vi "test_display.vi"() -> ()   [LabVIEW 2016]
uses:
  <vilib>/Utility/miscctls.llb/LVBoundsTypeDef.ctl
panel:
  out "Bounds":T1
  in  "[user-specified font]":T2={"Font Name:"="", "Size"=12, "Strikeout?"=FALSE, "Italic?"=FALSE, "Underline?"=FALSE, "Outline?"=FALSE, "Shadow?"=FALSE, "Bold?"=FALSE}
  in  "desired font(Application)":T3(ring)=enum."Application Font"
  in  "OK Button":bool
  in  "stop":bool
  out "text":string
  in  "origin":cluster{"x":i16, "y":i16}
  in  "alignment":T4
  out "2D Picture":picture
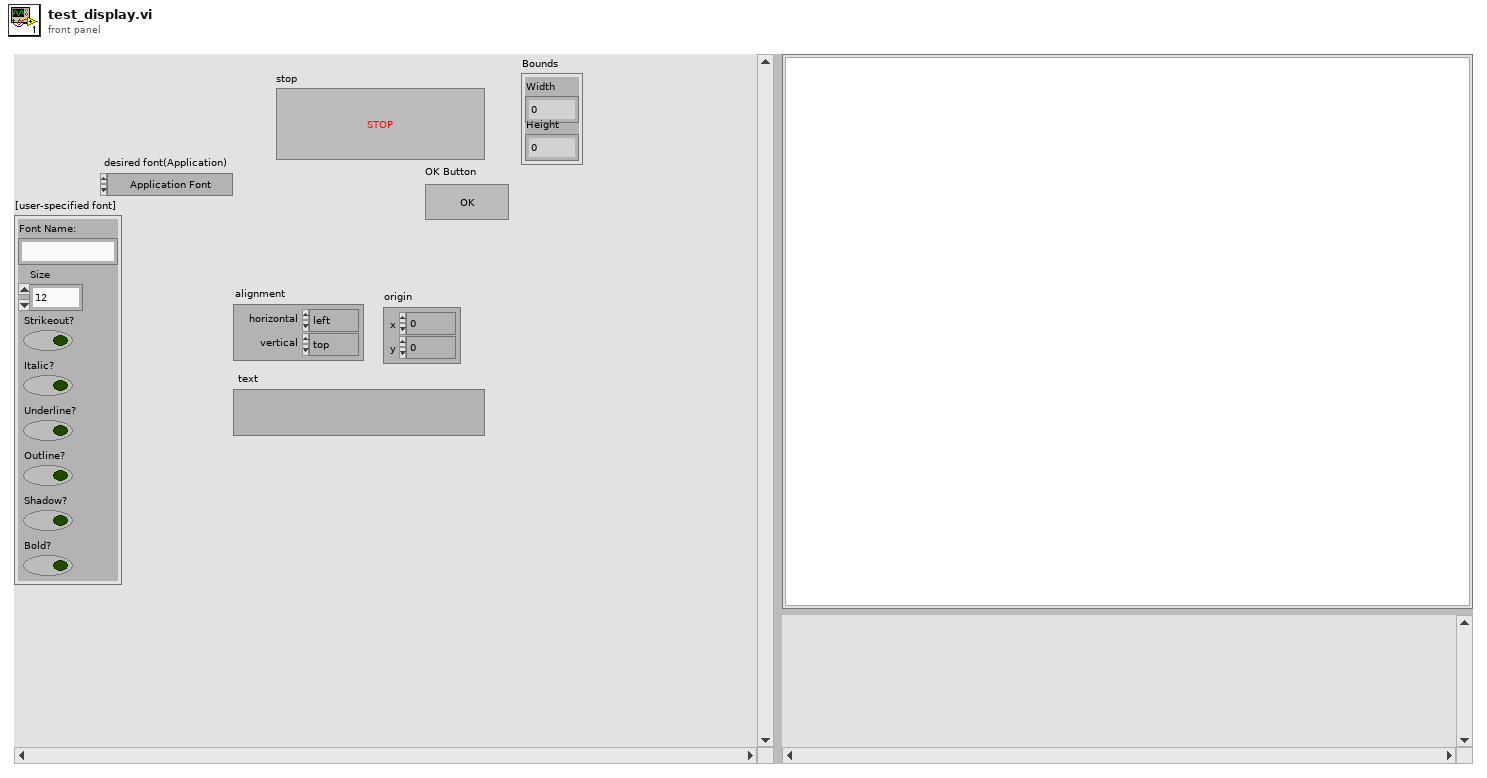
[diagram p1: front panel]
types:
  T1 = typedef "LVBoundsTypeDef.ctl" = cluster{"Width":u32, "Height":u32}
  T2 = cluster{"Font Name:":string, "Size":i16, "Strikeout?":bool, "Italic?":bool, "Underline?":bool, "Outline?":bool, "Shadow?":bool, "Bold?":bool}
  T3 = enum16{"User-specified Font", "Application Font", "System Font", "Dialog Font"}
  T4 = cluster{"horizontal":enum16{"left", "center", "right"}, "vertical":enum16{"top", "center", "bottom"}}
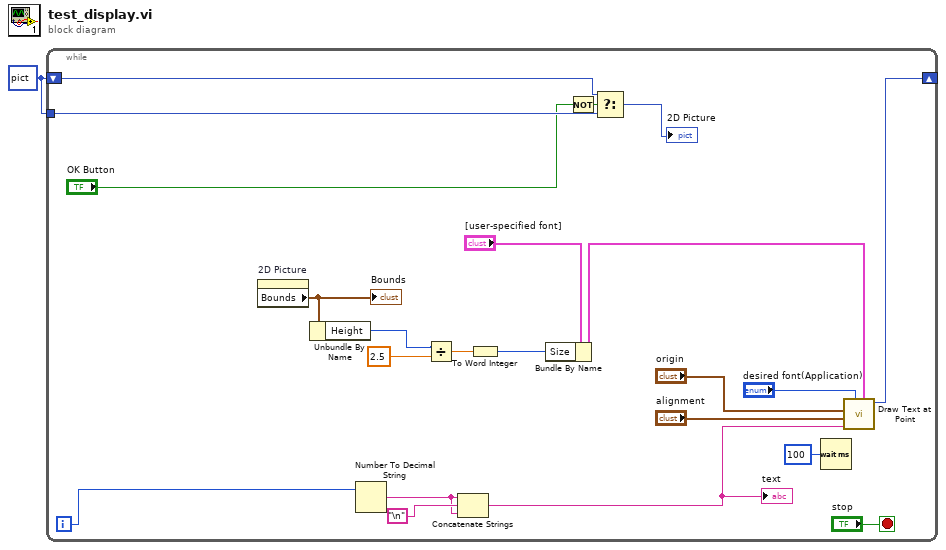
[diagram p0: block diagram]
diagram:
  w1 = picture data[5B] ("new picture")
  n1 = while {
    shift-right: [w23] -> _
    shift-left: w1 -> [w18]
    tunnel: w1 -> [w17]
    i -> [w11]
    stop <- "stop" stop-if-true
    n2 = property on="2D Picture" class="Pict"() -> ("Bounds"=w10:T1)  [unwired: 2 in, 2 out]
    "Bounds" <- w10
    n3 = Unbundle By Name(w10) -> ("Height"=w9:u32)
    n4 = Number To Decimal String(number=w11) -> (decimal integer string=w2:string)  [unwired: 1 in]
    n5 = Divide(x=w9, y=2.5) -> (x/y=w7:dbl)
    n6 = Concatenate Strings(w2, "\n", w2) -> (w4:string)
    "text" <- w4
    n7 = To Word Integer(number=w7) -> (16bit integer=w5:i16)
    n8 = Bundle By Name(cluster="[user-specified font]", "Size"=w5) -> (w6:T2)
    n9 = Not(x="OK Button") -> (.not. x?=w14:bool)
    n10 = Select(t=w18, s=w14, f=w17) -> (s? t:f=→"2D Picture":picture)
    n11 = Wait (ms)(milliseconds to wait=u32 100) -> ()  [unwired: 1 out]
    n12 = call <vilib>:"Draw Text at Point.vi"("[user-specified font]"=w6, "desired font(Application)"="desired font(Application)", "text"=w4, "alignment(left, top)"="alignment", "origin"="origin") -> ("new picture"=w23:picture)  [unwired: 5 in, 1 out]
  }
